vi "SubVI FM Demodulation Complex to Polar WF.vi"(0 "输入信号":waveform(cdb)) -> (1 "相角":waveform(dbl), 2 "幅值":waveform(dbl))   [LabVIEW 2015]
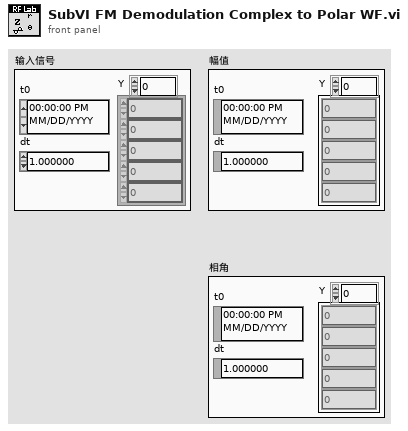
[diagram p1: front panel]
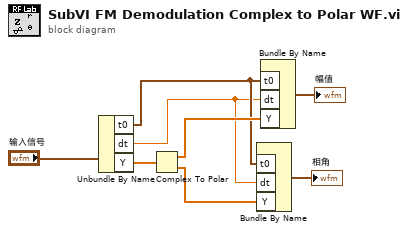
[diagram p0: block diagram]
diagram:
  n1 = Unbundle By Name("输入信号") -> ("t0"=w4:timestamp, "dt"=w3:dbl, "Y"=w7:cdb[])
  n2 = Complex To Polar(r * e^(i*theta)=w7) -> (r=w6:dbl[], theta=w5:dbl[])
  n3 = Bundle By Name("t0"=w4, "dt"=w3, "Y"=w5) -> (→"相角":waveform(dbl))  [unwired: 1 in]
  n4 = Bundle By Name("t0"=w4, "dt"=w3, "Y"=w6) -> (→"幅值":waveform(dbl))  [unwired: 1 in]
